vi "MegaAwesome_8_29_12b_JW.vi"() -> ()   [LabVIEW 2011]
uses:
  MegaAwesome_States.ctl
panel:
  out "Folder Index":i32 caption="Length"
  out "Image Preview":T1(plugin-control)
  out "Sat Id-Used":dbl[](array[numeric])
  out "Sat Vg Array-Used":dbl[](array[numeric])
  out "Vg Array-Log-Used":dbl[](array[numeric])
  out "Sat Id-Log-Used":dbl[](array[numeric])
  out "Lin Id-Used":dbl[](array[numeric])
  out "Lin-Vg Array-Used":dbl[](array[numeric])
  out "Lin Vd":dbl
  out "Recorded Prop":T2
  out "Current State":T3
  in  "Main Tab Control":T4(tab)
  in  "Image Folder":path
  out "Image File":path=path "D:/UserData/Desktop/Jeremy/WFU/Research/Programs/VI mods/Image Not Found.png"
  in  "Transfer File":path
  out "Transfer Folder":path
  out "Fabrication Prop":T5
  in  "File Controls":T6
  out "Date Recorded":string="Date Recorded" caption="Measured"
  out "Data Name:":string
  out "Image Name":string
  out "Index":string
  out "Date Created":string caption="Fabricated"
  in  "Comments:":string
  out "Rec: Length":dbl caption="Length" format="%#_3g"
  out "Rec: Width":dbl caption="Width" format="%#_4g"
  out "Rec: Dielectric (d)":dbl caption="Dielectric (d)" format="%#_3g"
  in  "New: Dielectric":dbl
  in  "New: Length":dbl
  in  "New: Width":dbl
  out "Rec: Temp":dbl caption="Sample Temp" format="%.1f"
  in  "New: Temp":dbl format="%.1f"
  in  "Independant Variable":string(combo)="Length (um):"
  out "Image Out":T1(plugin-control)
  in  "Num Pts":dbl=5.0
  in  "Num Pts Log":dbl=5.0 caption="Num Pts"
  out "Recorded Values Cluster":T7
  out "Calculated Values Cluster":T7 caption="Recorded Values Cluster"
  out "Re-Calculated Values Cluster":T7 caption="Recorded Values Cluster"
  in  "Origin Project File":path=path "\\\\acad1\\physics/Jurchescu-group/JW-PD/Group Library/Origin Project Files/DeviceData_8_10_12a_JW.opj"
  in  "No Image File":path=path "\\\\acad1\\physics/Jurchescu-group/JW-PD/Mega Awesome/Image Not Found.png"
  in  "Room Temp":dbl=294.0
  # "Image Location"
  # "Recorded"
  # "Calculated"
  # "Re-Calculated"
  # "Manual"
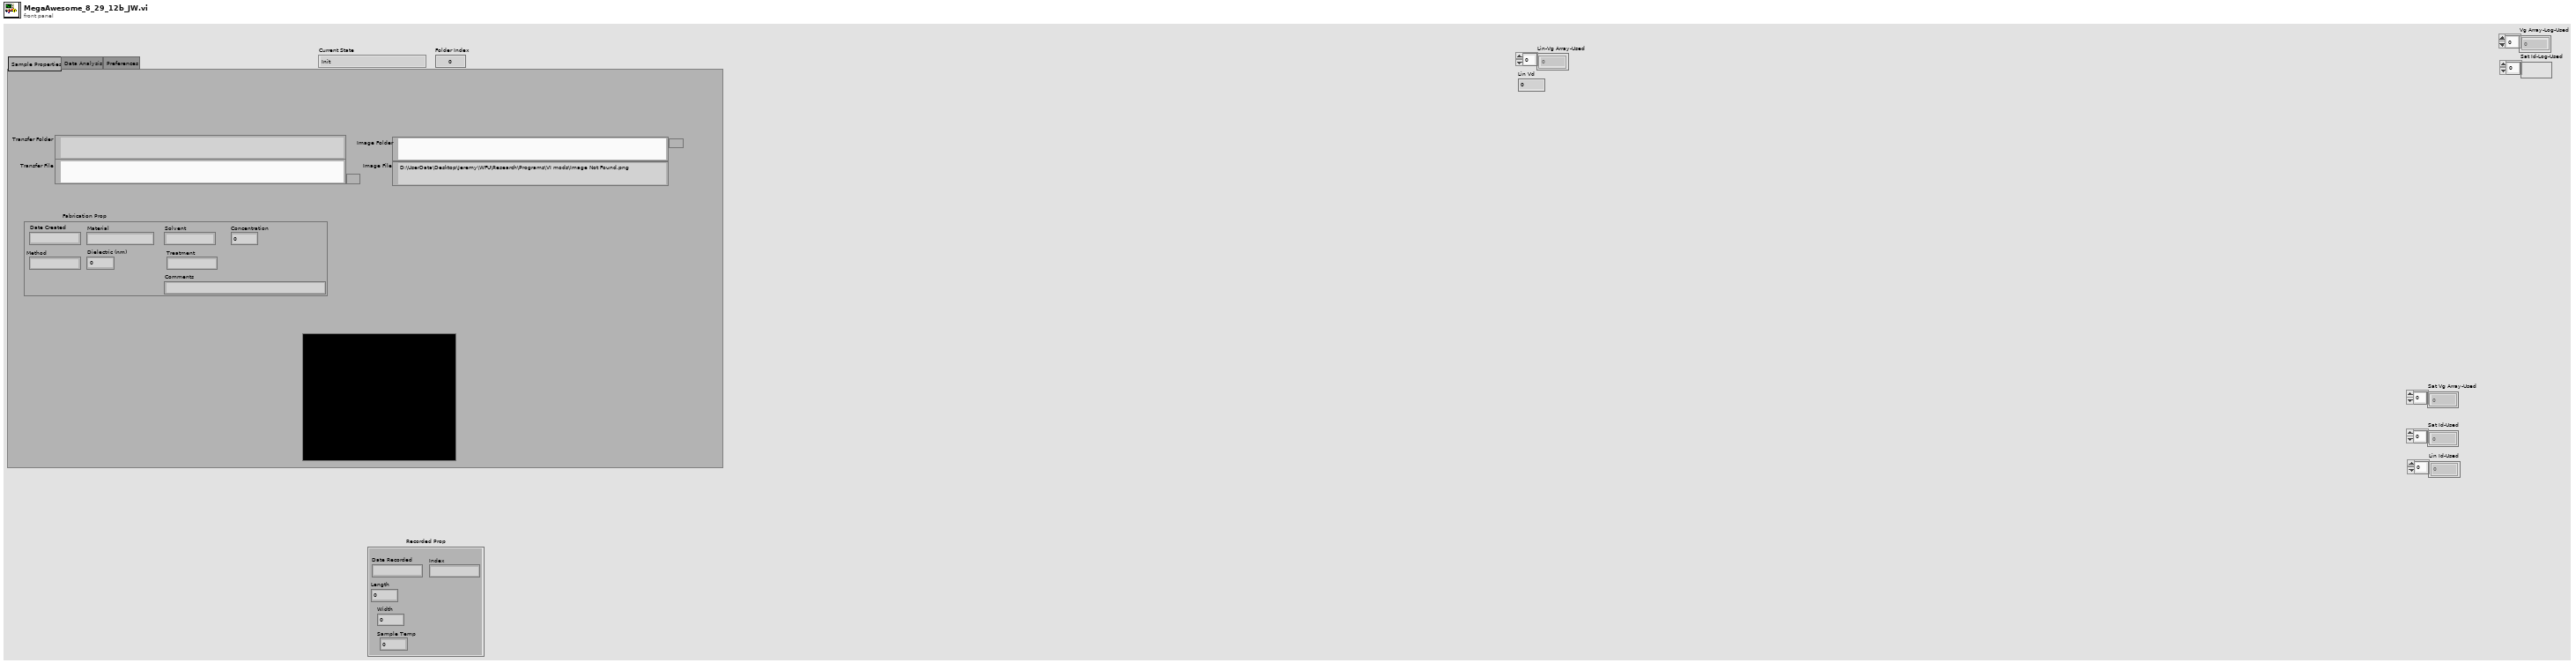
[diagram p1: front panel]
types:
  T1 = typedef "IMAQ Image.ctl" = refnum<image>
  T2 = cluster{"Date Recorded":string, "Index":string, "Length":dbl, "Width":dbl, "Sample Temp":dbl}
  T3 = typedef "MegaAwesome_States.ctl" = enum16{"Init", "File Missing", "No Event", "Read Data", "Calculated Values", "Re-Calculated Values", "Next File", "Previous File", "Discard File", "Save", "Save Lines", "Export", "Exit"}
  T4 = enum32{"Sample Properties", "Data Analysis", "Preferences"}
  T5 = cluster{"Date Created":string, "Material":string, "Solvent":string, "Concentration":dbl, "Method":string, "Dielectric (nm)":dbl, "Treatment":string, "Comments":string}
  T6 = cluster{"Previous File":bool, "Discard ":bool, "Save Lines":bool, "Close":bool, "Next File ":bool, "Save":bool, "Save Next":bool, "Export":bool}
  T7 = cluster{"Mobility-Sat":dbl, "Moblitity-Lin":dbl, "On/Off":dbl, "Off Current":dbl, "Vt-Sat":dbl, "STS":dbl, "Trap Density-VT":dbl, "Trap Density-STS":dbl}
  T8 = cluster{"Mobility-Sat":dbl, "Vt-Sat":dbl, "Mobility-Lin":dbl, "Vt-Lin":dbl, "Off I-Sat":dbl, "On/Off I-Sat":dbl}
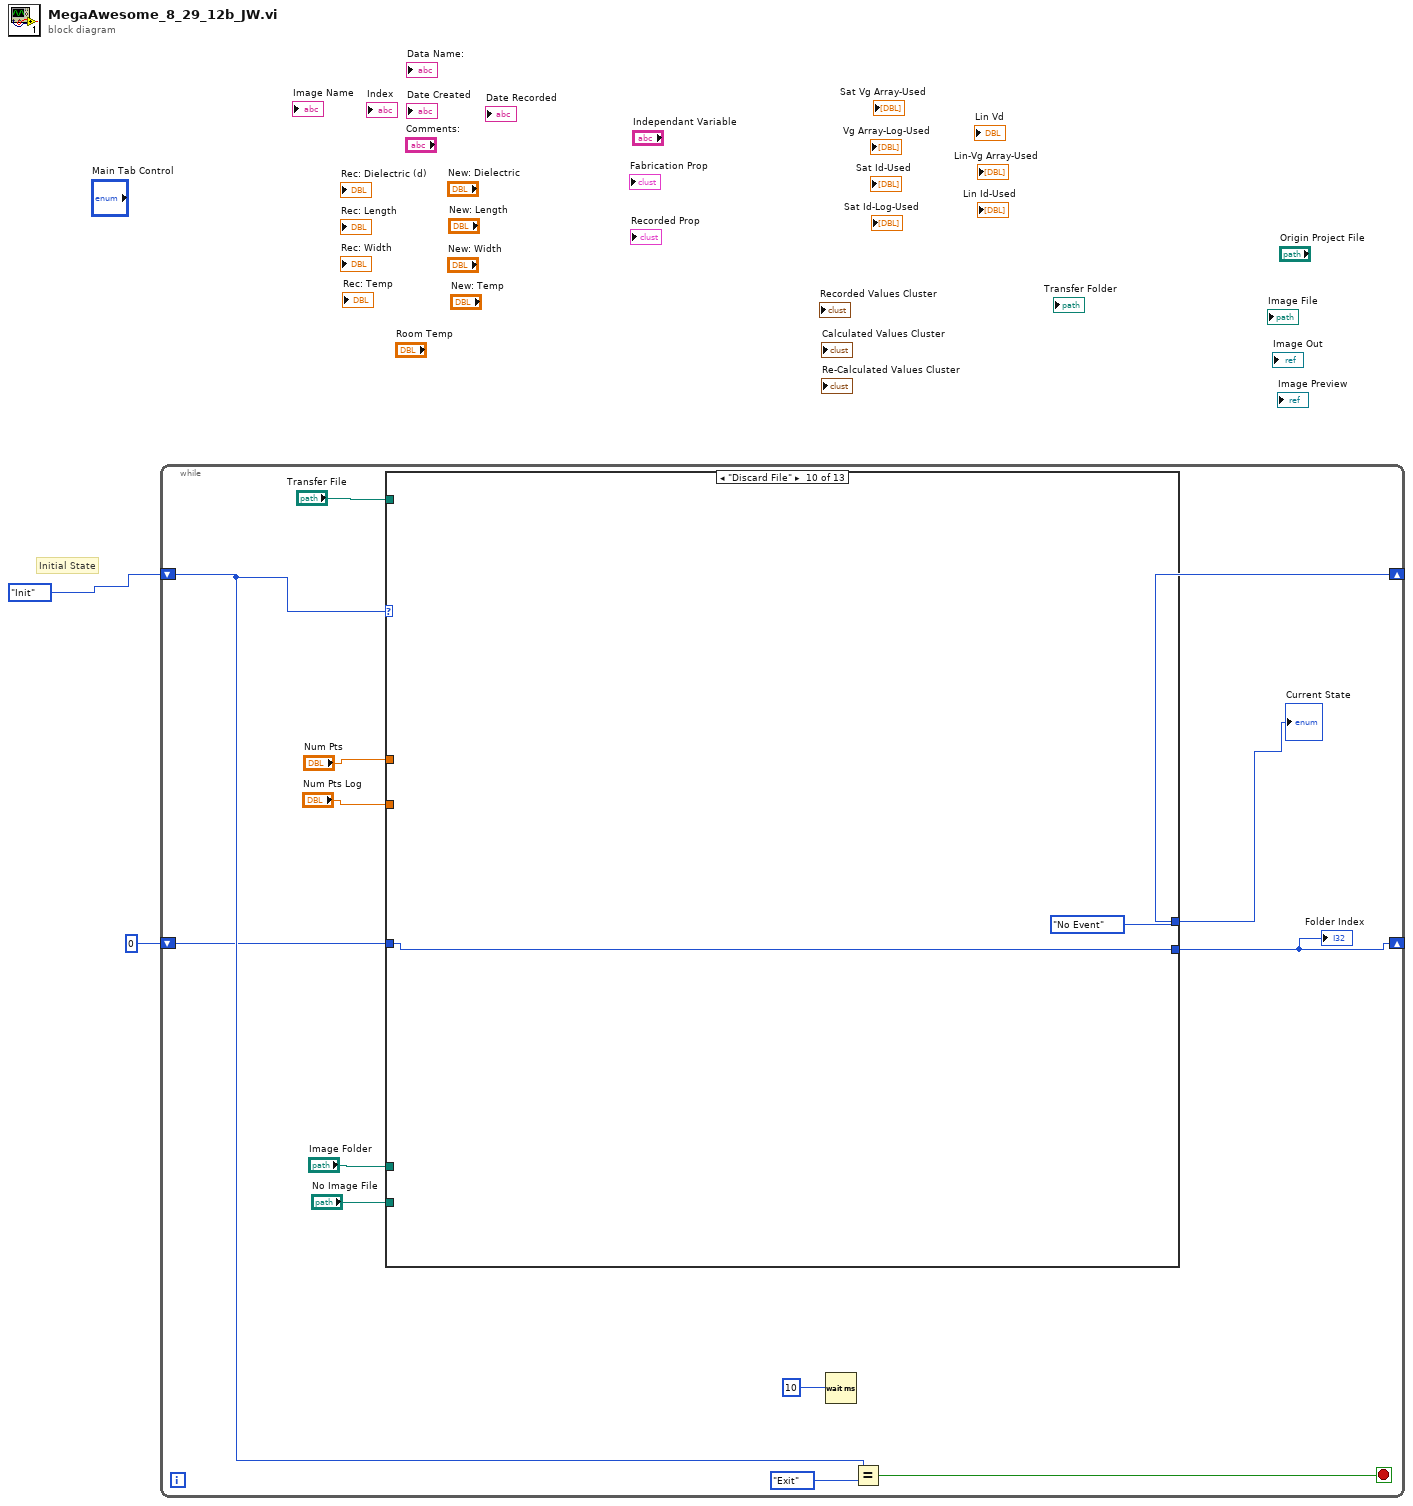
[diagram p0: block diagram]
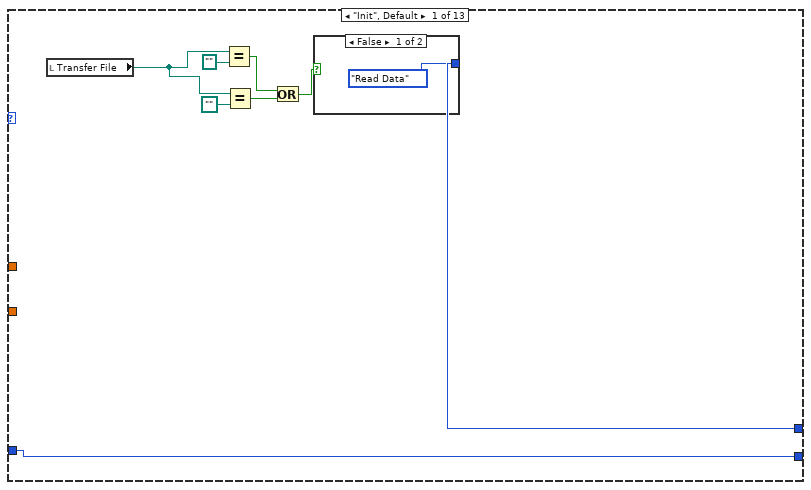
[diagram p2: hidden frame]
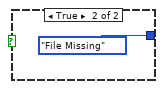
[diagram p3: hidden frame]
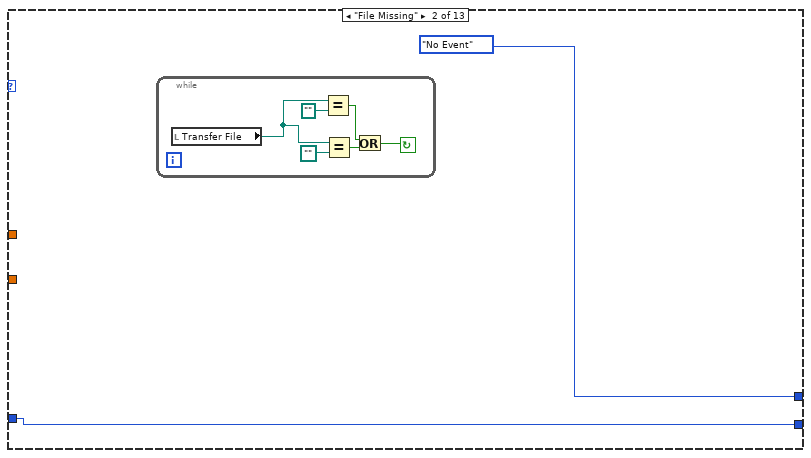
[diagram p4: hidden frame]
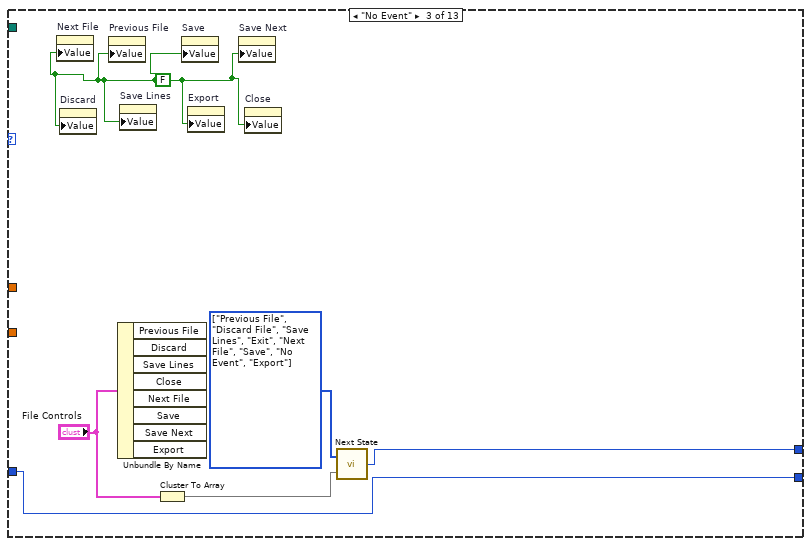
[diagram p5: hidden frame]
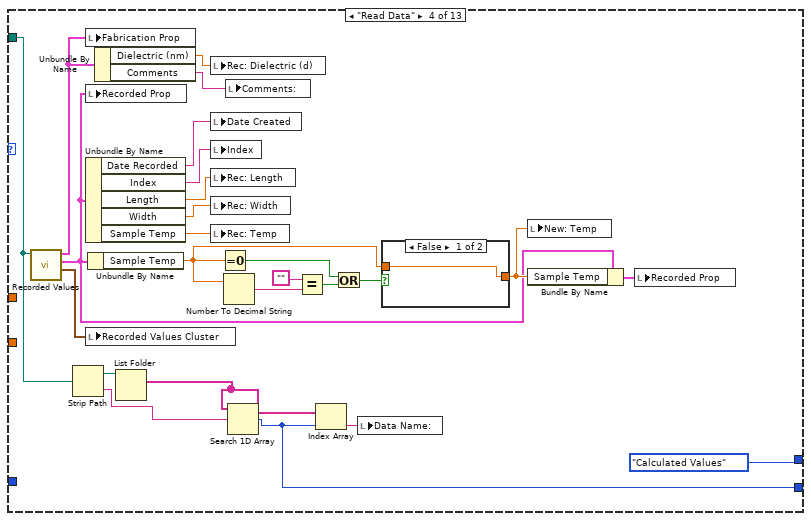
[diagram p6: hidden frame]
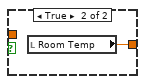
[diagram p7: hidden frame]
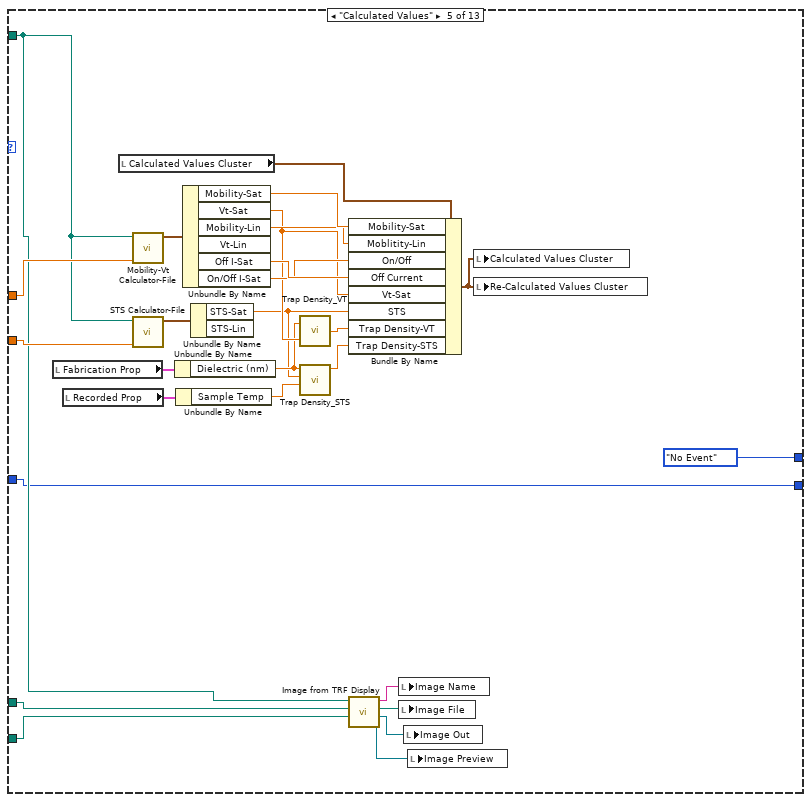
[diagram p8: hidden frame]
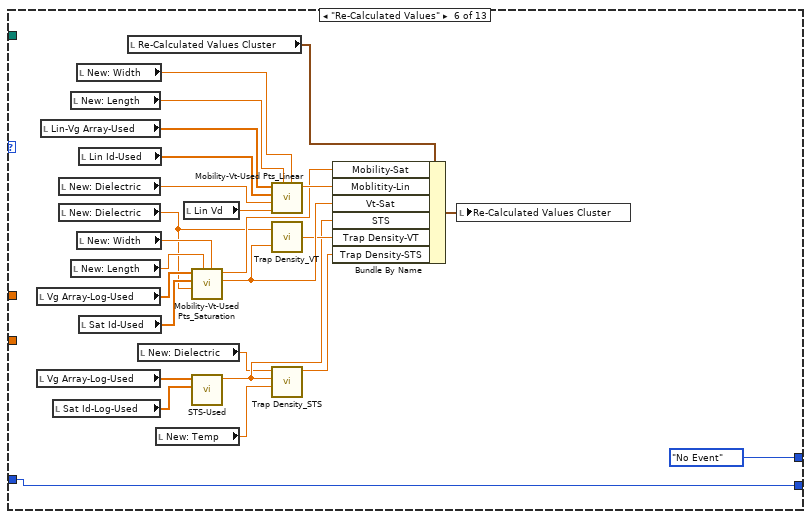
[diagram p9: hidden frame]
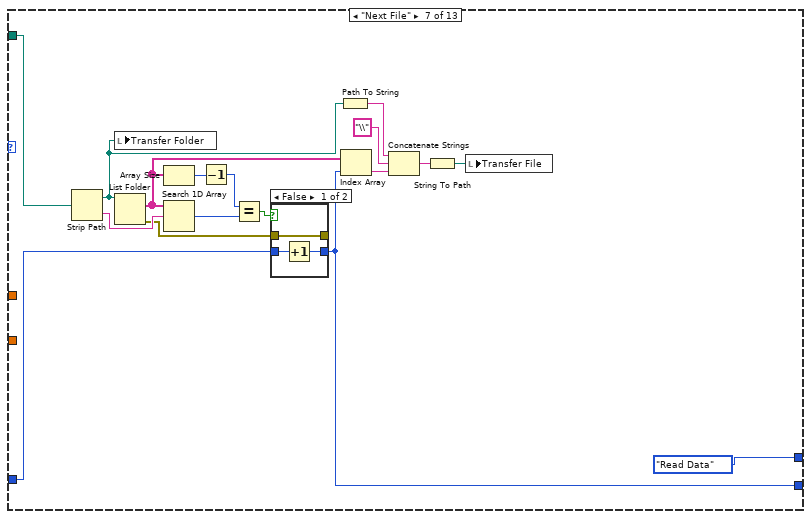
[diagram p10: hidden frame]
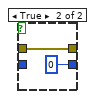
[diagram p11: hidden frame]
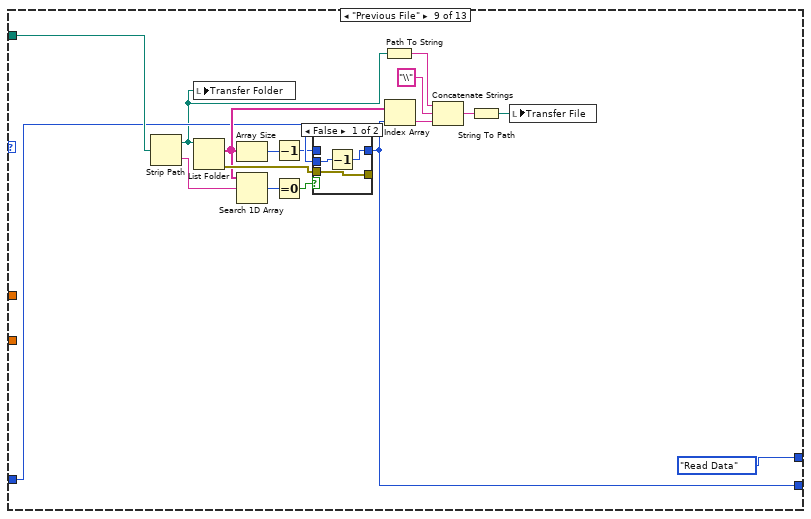
[diagram p13: hidden frame]
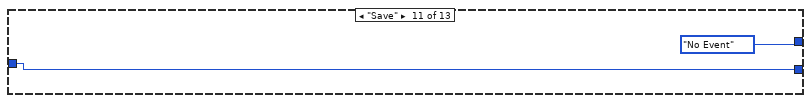
[diagram p15: hidden frame]
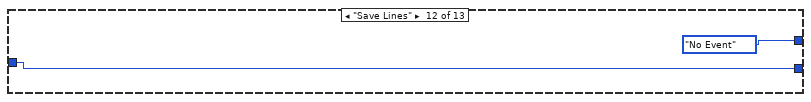
[diagram p16: hidden frame]
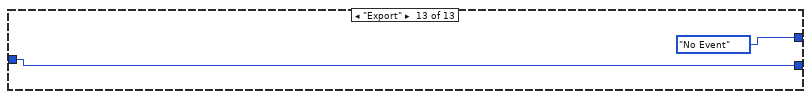
[diagram p17: hidden frame]
diagram:
  # "Initial State"
  n1 = while {
    shift-right: [w11] -> _
    shift-left: MegaAwesome_States."Init" -> [w13]
    shift-right: [w4] -> _
    shift-left: 0 -> [w5]
    stop <- w14 stop-if-true
    n2 = case shown="\"Discard File\"" w13 {
      selector: w13 -> [_ _ _ _ _ _ _ w141 _ _ _ _ _]
      tunnel: [w16 MegaAwesome_States."No Event" w36 MegaAwesome_States."Calculated Values" MegaAwesome_States."No Event" MegaAwesome_States."No Event" MegaAwesome_States."Read Data" w141 MegaAwesome_States."Read Data" MegaAwesome_States."No Event" MegaAwesome_States."No Event" MegaAwesome_States."No Event" MegaAwesome_States."No Event"] -> w11
      tunnel: "Transfer File" -> [_ _ _ w45 w73 _ w134 _ w148 _ _ _ _]
      tunnel: "Num Pts" -> [_ _ _ _ w77 _ _ _ _ _ _ _ _]
      tunnel: "Num Pts Log" -> [_ _ _ _ w76 _ _ _ _ _ _ _ _]
      tunnel: "Image Folder" -> [_ _ _ _ w72 _ _ _ _ _ _ _ _]
      tunnel: "No Image File" -> [_ _ _ _ w71 _ _ _ _ _ _ _ _]
      tunnel: [w15 w25 w33 w39 w66 w93 w119 w140 w146 w164 w166 w168 w170] -> w4
      tunnel: w5 -> [w15 w25 w33 _ w66 w93 w120 w140 w147 w164 w166 w168 w170]
      frame "Init", Default {
        n3 = local read "Transfer File"() -> (w17:path)
        n4 = Equal?(x=w17, y=path "") -> (x = y?=w20:bool)
        n5 = Equal?(x=w17, y=path "") -> (x = y?=w19:bool)
        n6 = Or(x=w20, y=w19) -> (x .or. y?=w22:bool)
        n7 = case shown="False" w22 {
          tunnel: [MegaAwesome_States."Read Data" MegaAwesome_States."File Missing"] -> w16
          frame False {
          }
          frame True {
          }
        }
      }
      frame "File Missing" {
        n8 = while {
          stop <- w27 continue-if-true
          n9 = local read "Transfer File"() -> (w28:path)
          n10 = Equal?(x=w28, y=path "") -> (x = y?=w30:bool)
          n11 = Equal?(x=w28, y=path "") -> (x = y?=w31:bool)
          n12 = Or(x=w30, y=w31) -> (x .or. y?=w27:bool)
        }
      }
      frame "No Event" {
        w37 = T3[] [enum."Previous File", enum."Discard File", enum."Save Lines", enum."Exit", enum."Next File", enum."Save", enum."No Event", enum."Export"] items=["Init", "File Missing", "No Event", "Read Data", "Calculated Values", "Re-Calculated Values", "Next File", "Previous File", "Discard File", "Save", "Save Lines", "Export", "Exit"]
        w38 = FALSE
        n13 = property on="Next File" class="Bool (strict)"("Value"=w38) -> ()  [unwired: 2 in, 2 out]
        n14 = property on="Discard" class="Bool (strict)"("Value"=w38) -> ()  [unwired: 2 in, 2 out]
        n15 = property on="Previous File" class="Bool (strict)"("Value"=w38) -> ()  [unwired: 2 in, 2 out]
        n16 = Unbundle By Name("File Controls") -> ()  [unwired: 8 out]
        n17 = property on="Save Lines" class="Bool (strict)"("Value"=w38) -> ()  [unwired: 2 in, 2 out]
        n18 = Cluster To Array(cluster="File Controls") -> (array=w34:bool[])
        n19 = property on="Save" class="Bool (strict)"("Value"=w38) -> ()  [unwired: 2 in, 2 out]
        n20 = property on="Export" class="Bool (strict)"("Value"=w38) -> ()  [unwired: 2 in, 2 out]
        n21 = property on="Save Next" class="Bool (strict)"("Value"=w38) -> ()  [unwired: 2 in, 2 out]
        n22 = property on="Close" class="Bool (strict)"("Value"=w38) -> ()  [unwired: 2 in, 2 out]
        n23 = call "Next State.vi"("Buttons []"=w34, "States []"=w37) -> ("Enum"=w36:T3)
      }
      frame "Read Data" {
        n24 = call "Recorded Values.vi"("Path"=w45) -> ("Recorded Char"=w63:T7, "Recorded Prop"=w53:T2, "Fabrication Prop"=w47:T5)  [unwired: 8 in]
        n25 = Strip Path(path=w45) -> (stripped path=w46:path, name=w44:string)
        n26 = local write "Fabrication Prop"(w47) -> ()
        n27 = local write "Recorded Prop"(w53) -> ()
        n28 = Unbundle By Name(w53) -> ("Date Recorded"=w52:string, "Index"=w50:string, "Length"=w51:dbl, "Width"=w49:dbl, "Sample Temp"=w48:dbl)
        n29 = local write "Recorded Values Cluster"(w63) -> ()
        n30 = Unbundle By Name(w53) -> ("Sample Temp"=w56:dbl)
        n31 = Unbundle By Name(w47) -> ("Dielectric (nm)"=w41:dbl, "Comments"=w40:string)
        n32 = List Folder(path=w46) -> (filenames=w42:string[])  [unwired: 3 in, 3 out]
        n33 = local write "Rec: Dielectric (d)"(w41) -> ()
        n34 = local write "Date Created"(w52) -> ()
        n35 = local write "Index"(w50) -> ()
        n36 = local write "Rec: Length"(w51) -> ()
        n37 = local write "Rec: Width"(w49) -> ()
        n38 = local write "Rec: Temp"(w48) -> ()
        n39 = Equal To 0?(x=w56) -> (x = 0?=w59:bool)
        n40 = Number To Decimal String(number=w56) -> (decimal integer string=w60:string)  [unwired: 1 in]
        n41 = local write "Comments:"(w40) -> ()
        n42 = Search 1D Array(1D array=w42, element=w44) -> (index of element=w39:i32)  [unwired: 1 in]
        n43 = Equal?(x="", y=w60) -> (x = y?=w58:bool)
        n44 = Index Array(array=w42, index=w39) -> (element=w43:string)
        n45 = Or(x=w59, y=w58) -> (x .or. y?=w57:bool)
        n46 = local write "Data Name:"(w43) -> ()
        n47 = case shown="False" w57 {
          tunnel: [w64 w65] -> w54
          tunnel: w56 -> [w64 _]
          frame False {
          }
          frame True {
            n48 = local read "Room Temp"() -> (w65:dbl)
          }
        }
        n49 = local write "New: Temp"(w54) -> ()
        n50 = Bundle By Name(cluster=w53, "Sample Temp"=w54) -> (w55:T2)
        n51 = local write "Recorded Prop"(w55) -> ()
      }
      frame "Calculated Values" {
        n52 = local read "Fabrication Prop"() -> (w82:T5)
        n53 = local read "Recorded Prop"() -> (w75:T2)
        n54 = local read "Calculated Values Cluster"() -> (w92:T7)
        n55 = call "Mobility-Vt Calculator-File.vi"("NumPts"=w77, "Path"=w73) -> ("Output"=w90:T8)  [unwired: 5 in, 4 out]
        n56 = call "STS Calculator-File.vi"("NumPts"=w76, "Path"=w73) -> ("Ouput"=w85:cluster{"STS-Sat":dbl, "STS-Lin":dbl})  [unwired: 5 in, 4 out]
        n57 = Unbundle By Name(w82) -> ("Dielectric (nm)"=w80:dbl)
        n58 = Unbundle By Name(w75) -> ("Sample Temp"=w74:dbl)
        n59 = Unbundle By Name(w90) -> ("Mobility-Sat"=w89:dbl, "Vt-Sat"=w81:dbl, "Mobility-Lin"=w88:dbl, "Off I-Sat"=w87:dbl, "On/Off I-Sat"=w86:dbl)  [unwired: 1 out]
        n60 = Unbundle By Name(w85) -> ("STS-Sat"=w79:dbl)  [unwired: 1 out]
        n61 = call "Trap Density_VT.vi"("VT"=w81, "Dielectric"=w80) -> ("Trap Density-VT"=w84:dbl)
        n62 = call "Trap Density_STS.vi"("Temp (T) [K]"=w74, "S.T.S. (S)"=w79, "Dielectric"=w80) -> ("Trap Density (N)"=w83:dbl)  [unwired: 8 in]
        n63 = Bundle By Name(cluster=w92, "Mobility-Sat"=w89, "Moblitity-Lin"=w88, "On/Off"=w86, "Off Current"=w87, "Vt-Sat"=w81, "STS"=w79, "Trap Density-VT"=w84, "Trap Density-STS"=w83) -> (w91:T7)
        n64 = call "Image from TRF Display.vi"("No Image File"=w71, "Image Folder"=w72, "Transfer File"=w73) -> ("Image Out 2"=w67:T1, "Image Out"=w68:T1, "Image File"=w69:path, "Image Name"=w70:string)  [unwired: 5 in]
        n65 = local write "Image Name"(w70) -> ()
        n66 = local write "Image File"(w69) -> ()
        n67 = local write "Image Out"(w68) -> ()
        n68 = local write "Image Preview"(w67) -> ()
        n69 = local write "Calculated Values Cluster"(w91) -> ()
        n70 = local write "Re-Calculated Values Cluster"(w91) -> ()
      }
      frame "Re-Calculated Values" {
        n71 = local read "Vg Array-Log-Used"() -> (w108:dbl[])
        n72 = local read "Vg Array-Log-Used"() -> (w100:dbl[])
        n73 = local read "Lin-Vg Array-Used"() -> (w115:dbl[])
        n74 = local read "Sat Id-Log-Used"() -> (w99:dbl[])
        n75 = local read "New: Dielectric"() -> (w113:dbl)
        n76 = local read "New: Dielectric"() -> (w97:dbl)
        n77 = local read "New: Length"() -> (w111:dbl)
        n78 = local read "New: Length"() -> (w107:dbl)
        n79 = local read "New: Width"() -> (w110:dbl)
        n80 = local read "New: Width"() -> (w106:dbl)
        n81 = local read "Lin Id-Used"() -> (w114:dbl[])
        n82 = local read "Sat Id-Used"() -> (w105:dbl[])
        n83 = local read "Re-Calculated Values Cluster"() -> (w117:T7)
        n84 = local read "New: Dielectric"() -> (w96:dbl)
        n85 = local read "New: Temp"() -> (w95:dbl)
        n86 = local read "Lin Vd"() -> (w112:dbl)
        n87 = call "Mobility-Vt-Used Pts_Saturation.vi"("Width"=w106, "Length"=w107, "Dielectric (d)"=w97, "Sat Id Used"=w105, "Vg Used"=w108) -> ("Vt"=w103:dbl, "Mobility"=w104:dbl)  [unwired: 4 in, 1 out]
        n88 = call "STS-Used.vi"("Id Used"=w99, "Vg-Used"=w100) -> ("STS"=w98:dbl)  [unwired: 9 in]
        n89 = call "Mobility-Vt-Used Pts_Linear.vi"("Width"=w110, "Length"=w111, "Vd"=w112, "Dielectric (d)"=w113, "Sat Id Used"=w114, "Vg Used"=w115) -> ("Mobility"=w109:dbl)  [unwired: 3 in, 2 out]
        n90 = call "Trap Density_VT.vi"("VT"=w103, "Dielectric"=w97) -> ("Trap Density-VT"=w102:dbl)
        n91 = call "Trap Density_STS.vi"("Temp (T) [K]"=w95, "S.T.S. (S)"=w98, "Dielectric"=w96) -> ("Trap Density (N)"=w94:dbl)  [unwired: 8 in]
        n92 = Bundle By Name(cluster=w117, "Mobility-Sat"=w104, "Moblitity-Lin"=w109, "Vt-Sat"=w103, "STS"=w98, "Trap Density-VT"=w102, "Trap Density-STS"=w94) -> (w116:T7)
        n93 = local write "Re-Calculated Values Cluster"(w116) -> ()
      }
      frame "Next File" {
        n94 = Strip Path(path=w134) -> (stripped path=w124:path, name=w132:string)
        n95 = local write "Transfer Folder"(w124) -> ()
        n96 = List Folder(path=w124) -> (filenames=w118:string[], error out=w127:errorcluster)  [unwired: 3 in, 2 out]
        n97 = Array Size(array=w118) -> (size(s)=w131:i32)
        n98 = Search 1D Array(1D array=w118, element=w132) -> (index of element=w129:i32)  [unwired: 1 in]
        n99 = Decrement(x=w131) -> (x-1=w130:i32)
        n100 = Equal?(x=w130, y=w129) -> (x = y?=w128:bool)
        n101 = case shown="False" w128 {
          tunnel: w120 -> [w137 _]
          tunnel: [w136 0] -> w119
          tunnel: w127 -> [w135 w138]
          tunnel: [w135 w138] -> _
          frame False {
            n102 = Increment(x=w137) -> (x+1=w136:i32)
          }
          frame True {
          }
        }
        n103 = Path To String(path=w124) -> (string=w125:string)
        n104 = Index Array(array=w118, index=w119) -> (element=w126:string)
        n105 = Concatenate Strings(w125, "\\", w126) -> (w122:string)
        n106 = String To Path(string=w122) -> (path=w121:path)
        n107 = local write "Transfer File"(w121) -> ()
      }
      frame "Exit" {
      }
      frame "Previous File" {
        n108 = Strip Path(path=w148) -> (stripped path=w145:path, name=w157:string)
        n109 = local write "Transfer Folder"(w145) -> ()
        n110 = List Folder(path=w145) -> (filenames=w149:string[], error out=w154:errorcluster)  [unwired: 3 in, 2 out]
        n111 = Array Size(array=w149) -> (size(s)=w143:i32)
        n112 = Search 1D Array(1D array=w149, element=w157) -> (index of element=w156:i32)  [unwired: 1 in]
        n113 = Decrement(x=w143) -> (x-1=w142:i32)
        n114 = Equal To 0?(x=w156) -> (x = 0?=w155:bool)
        n115 = case shown="False" w155 {
          tunnel: w147 -> [w161 _]
          tunnel: [w160 w162] -> w146
          tunnel: w154 -> [w159 w163]
          tunnel: [w159 w163] -> _
          tunnel: w142 -> [_ w162]
          frame False {
            n116 = Decrement(x=w161) -> (x-1=w160:i32)
          }
          frame True {
          }
        }
        n117 = Path To String(path=w145) -> (string=w144:string)
        n118 = Index Array(array=w149, index=w146) -> (element=w153:string)
        n119 = Concatenate Strings(w144, "\\", w153) -> (w151:string)
        n120 = String To Path(string=w151) -> (path=w150:path)
        n121 = local write "Transfer File"(w150) -> ()
      }
      frame "Discard File" {
      }
      frame "Save" {
      }
      frame "Save Lines" {
      }
      frame "Export" {
      }
    }
    "Current State" <- w11
    "Folder Index" <- w4
    n122 = Wait (ms)(milliseconds to wait=10) -> ()  [unwired: 1 out]
    n123 = Equal?(x=w13, y=MegaAwesome_States."Exit") -> (x = y?=w14:bool)
  }
